vi "Terminal-GearSystem-Getter20150815.vi"(8 "error in (no error)":errorcluster caption="错误输入（无错误）", 11 "read operation timeout (ms)":i32=5000 caption="读操作超时（5000毫秒）") -> (0 "error out":errorcluster caption="错误输出", 2 "时间标识":timestamp, 3 "设备信息":T1)   [LabVIEW 2014]
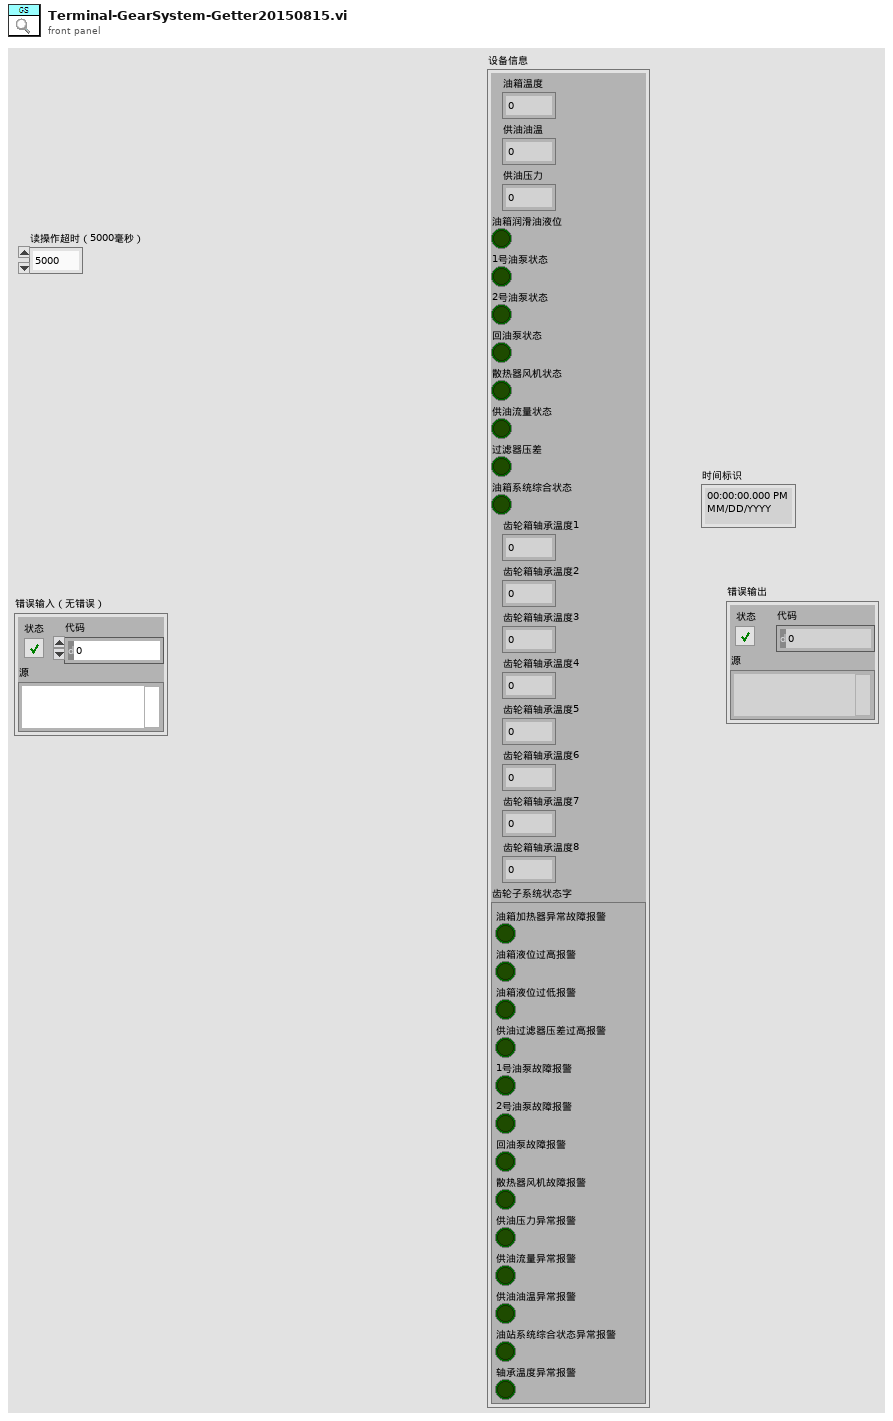
[diagram p1: front panel]
types:
  T1 = cluster{"油箱温度":u16, "供油油温":u16, "供油压力":u16, "油箱润滑油液位":bool, "1号油泵状态":bool, "2号油泵状态":bool, "回油泵状态":bool, "散热器风机状态":bool, "供油流量状态":bool, "过滤器压差":bool, "油箱系统综合状态":bool, "齿轮箱轴承温度1":u16, "齿轮箱轴承温度2":u16, "齿轮箱轴承温度3":u16, "齿轮箱轴承温度4":u16, "齿轮箱轴承温度5":u16, "齿轮箱轴承温度6":u16, "齿轮箱轴承温度7":u16, "齿轮箱轴承温度8":u16, "齿轮子系统状态字":cluster{"油箱加热器异常故障报警":bool, "油箱液位过高报警":bool, "油箱液位过低报警":bool, "供油过滤器压差过高报警":bool, "1号油泵故障报警":bool, "2号油泵故障报警":bool, "回油泵故障报警":bool, "散热器风机故障报警":bool, "供油压力异常报警":bool, "供油流量异常报警":bool, "供油油温异常报警":bool, "油站系统综合状态异常报警":bool, "轴承温度异常报警":bool}}
  T2 = cluster{"油箱温度":u16, "供油油温":u16, "供油压力":u16, "油箱润滑油液位":u16, "1号油泵状态":u16, "2号油泵状态":u16, "回油泵状态":u16, "散热器风机状态":u16, "供油流量状态":u16, "过滤器压差":u16, "油箱系统综合状态":u16, "齿轮箱轴承温度1":u16, "齿轮箱轴承温度2":u16, "齿轮箱轴承温度3":u16, "齿轮箱轴承温度4":u16, "齿轮箱轴承温度5":u16, "齿轮箱轴承温度6":u16, "齿轮箱轴承温度7":u16, "齿轮箱轴承温度8":u16, "齿轮子系统状态字":cluster{"油箱加热器异常故障报警":bool, "油箱液位过高报警":bool, "油箱液位过低报警":bool, "供油过滤器压差过高报警":bool, "1号油泵故障报警":bool, "2号油泵故障报警":bool, "回油泵故障报警":bool, "散热器风机故障报警":bool, "供油压力异常报警":bool, "供油流量异常报警":bool, "供油油温异常报警":bool, "油站系统综合状态异常报警":bool, "轴承温度异常报警":bool}}
  T3 = cluster{"油箱加热器异常故障报警":bool, "油箱液位过高报警":bool, "油箱液位过低报警":bool, "供油过滤器压差过高报警":bool, "1号油泵故障报警":bool, "2号油泵故障报警":bool, "回油泵故障报警":bool, "散热器风机故障报警":bool, "供油压力异常报警":bool, "供油流量异常报警":bool, "供油油温异常报警":bool, "油站系统综合状态异常报警":bool, "轴承温度异常报警":bool}
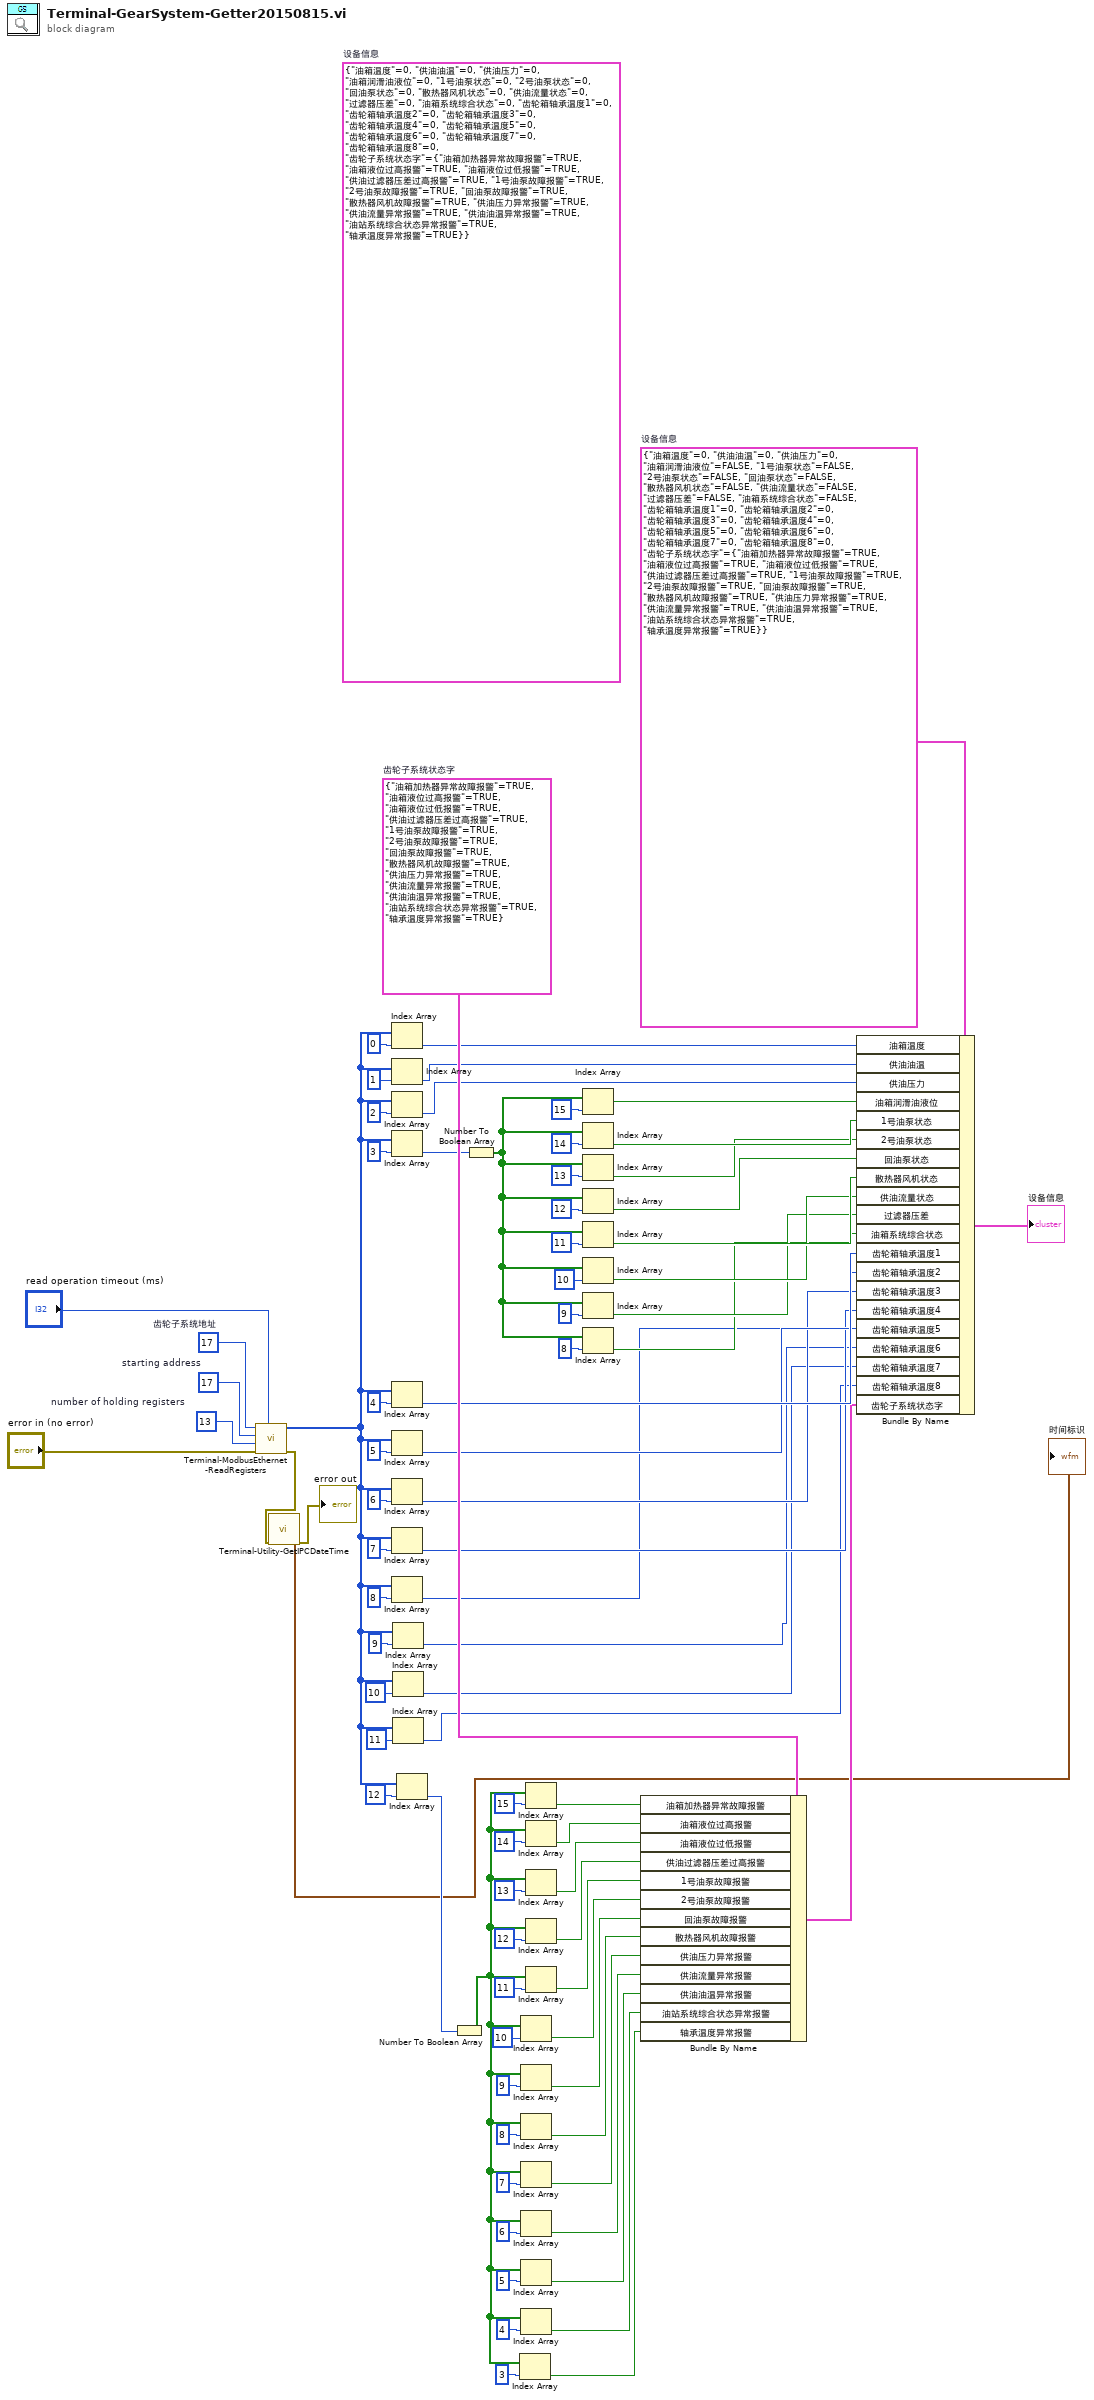
[diagram p0: block diagram]
diagram:
  (unwired) T2 {"油箱温度"=0, "供油油温"=0, "供油压力"=0, "油箱润滑油液位"=0, "1号油泵状态"=0, "2号油泵状态"=0, "回油泵状态"=0, "散热器风机状态"=0, "供油流量状态"=0, "过滤器压差"=0, "油箱系统综合状态"=0, "齿轮箱轴承温度1"=0, "齿轮箱轴承温度2"=0, "齿轮箱轴承温度3"=0, "齿轮箱轴承温度4"=0, "齿轮箱轴承温度5"=0, "齿轮箱轴承温度6"=0, "齿轮箱轴承温度7"=0, "齿轮箱轴承温度8"=0, "齿轮子系统状态字"={"油箱加热器异常故障报警"=TRUE, "油箱液位过高报警"=TRUE, "油箱液位过低报警"=TRUE, "供油过滤器压差过高报警"=TRUE, "1号油泵故障报警"=TRUE, "2号油泵故障报警"=TRUE, "回油泵故障报警"=TRUE, "散热器风机故障报警"=TRUE, "供油压力异常报警"=TRUE, "供油流量异常报警"=TRUE, "供油油温异常报警"=TRUE, "油站系统综合状态异常报警"=TRUE, "轴承温度异常报警"=TRUE}}  # 设备信息
  w42 = T3 {"油箱加热器异常故障报警"=TRUE, "油箱液位过高报警"=TRUE, "油箱液位过低报警"=TRUE, "供油过滤器压差过高报警"=TRUE, "1号油泵故障报警"=TRUE, "2号油泵故障报警"=TRUE, "回油泵故障报警"=TRUE, "散热器风机故障报警"=TRUE, "供油压力异常报警"=TRUE, "供油流量异常报警"=TRUE, "供油油温异常报警"=TRUE, "油站系统综合状态异常报警"=TRUE, "轴承温度异常报警"=TRUE}  # 齿轮子系统状态字
  w78 = T1 {"油箱温度"=0, "供油油温"=0, "供油压力"=0, "油箱润滑油液位"=FALSE, "1号油泵状态"=FALSE, "2号油泵状态"=FALSE, "回油泵状态"=FALSE, "散热器风机状态"=FALSE, "供油流量状态"=FALSE, "过滤器压差"=FALSE, "油箱系统综合状态"=FALSE, "齿轮箱轴承温度1"=0, "齿轮箱轴承温度2"=0, "齿轮箱轴承温度3"=0, "齿轮箱轴承温度4"=0, "齿轮箱轴承温度5"=0, "齿轮箱轴承温度6"=0, "齿轮箱轴承温度7"=0, "齿轮箱轴承温度8"=0, "齿轮子系统状态字"={"油箱加热器异常故障报警"=TRUE, "油箱液位过高报警"=TRUE, "油箱液位过低报警"=TRUE, "供油过滤器压差过高报警"=TRUE, "1号油泵故障报警"=TRUE, "2号油泵故障报警"=TRUE, "回油泵故障报警"=TRUE, "散热器风机故障报警"=TRUE, "供油压力异常报警"=TRUE, "供油流量异常报警"=TRUE, "供油油温异常报警"=TRUE, "油站系统综合状态异常报警"=TRUE, "轴承温度异常报警"=TRUE}}  # 设备信息
  w81 = u16 13  # number of holding registers
  w82 = u16 17  # starting address
  w83 = u8 17  # 齿轮子系统地址
  n1 = call "Terminal-ModbusEthernet-ReadRegisters.vi"("read operation timeout (ms)"="read operation timeout (ms)", "error in"="error in (no error)", "number of holding registers"=w81, "starting address"=w82, "unit ID"=w83) -> ("error out"=w2:errorcluster, "register values"=w17:u16[])  [unwired: 5 in]
  n2 = call "Terminal-Utility-GetIPCDateTime.vi"("error in (no error)"=w2) -> ("error out"=→"error out":errorcluster, "时间标识"=→"时间标识":timestamp)  [unwired: 9 in]
  n3 = Index Array(array=w17, index=0 ("索引")) -> (element=w41:u16)
  n4 = Index Array(array=w17, index=1 ("索引")) -> (element=w40:u16)
  n5 = Index Array(array=w17, index=2 ("索引")) -> (element=w39:u16)
  n6 = Index Array(array=w17, index=3 ("索引")) -> (element=w38:u16)
  n7 = Index Array(array=w17, index=4 ("索引")) -> (element=w16:u16)
  n8 = Index Array(array=w17, index=5 ("索引")) -> (element=w15:u16)
  n9 = Index Array(array=w17, index=6 ("索引")) -> (element=w14:u16)
  n10 = Index Array(array=w17, index=7 ("索引")) -> (element=w13:u16)
  n11 = Index Array(array=w17, index=8 ("索引")) -> (element=w12:u16)
  n12 = Index Array(array=w17, index=9 ("索引")) -> (element=w11:u16)
  n13 = Index Array(array=w17, index=10 ("索引")) -> (element=w10:u16)
  n14 = Index Array(array=w17, index=11 ("索引")) -> (element=w9:u16)
  n15 = Index Array(array=w17, index=12 ("索引")) -> (element=w73:u16)
  n16 = Number To Boolean Array(number=w73) -> (Boolean array=w7:bool[])
  n17 = Number To Boolean Array(number=w38) -> (Boolean array=w29:bool[])
  n18 = Index Array(array=w7, index=3 ("索引")) -> (element=w6:bool)
  n19 = Index Array(array=w7, index=10 ("索引")) -> (element=w49:bool)
  n20 = Index Array(array=w7, index=9 ("索引")) -> (element=w48:bool)
  n21 = Index Array(array=w7, index=8 ("索引")) -> (element=w47:bool)
  n22 = Index Array(array=w7, index=7 ("索引")) -> (element=w46:bool)
  n23 = Index Array(array=w7, index=6 ("索引")) -> (element=w43:bool)
  n24 = Index Array(array=w7, index=5 ("索引")) -> (element=w44:bool)
  n25 = Index Array(array=w7, index=4 ("索引")) -> (element=w45:bool)
  n26 = Index Array(array=w7, index=15 ("索引")) -> (element=w69:bool)
  n27 = Index Array(array=w7, index=14 ("索引")) -> (element=w68:bool)
  n28 = Index Array(array=w7, index=13 ("索引")) -> (element=w52:bool)
  n29 = Index Array(array=w7, index=12 ("索引")) -> (element=w51:bool)
  n30 = Index Array(array=w7, index=11 ("索引")) -> (element=w50:bool)
  n31 = Index Array(array=w29, index=15 ("索引")) -> (element=w28:bool)
  n32 = Index Array(array=w29, index=14 ("索引")) -> (element=w27:bool)
  n33 = Index Array(array=w29, index=13 ("索引")) -> (element=w26:bool)
  n34 = Index Array(array=w29, index=12 ("索引")) -> (element=w25:bool)
  n35 = Index Array(array=w29, index=11 ("索引")) -> (element=w24:bool)
  n36 = Index Array(array=w29, index=10 ("索引")) -> (element=w23:bool)
  n37 = Index Array(array=w29, index=9 ("索引")) -> (element=w22:bool)
  n38 = Index Array(array=w29, index=8 ("索引")) -> (element=w21:bool)
  n39 = Bundle By Name(cluster=w42, "油箱加热器异常故障报警"=w69, "油箱液位过高报警"=w68, "油箱液位过低报警"=w52, "供油过滤器压差过高报警"=w51, "1号油泵故障报警"=w50, "2号油泵故障报警"=w49, "回油泵故障报警"=w48, "散热器风机故障报警"=w47, "供油压力异常报警"=w46, "供油流量异常报警"=w43, "供油油温异常报警"=w44, "油站系统综合状态异常报警"=w45, "轴承温度异常报警"=w6) -> (w5:T3)
  n40 = Bundle By Name(cluster=w78, "油箱温度"=w41, "供油油温"=w40, "供油压力"=w39, "油箱润滑油液位"=w28, "1号油泵状态"=w27, "2号油泵状态"=w26, "回油泵状态"=w25, "散热器风机状态"=w24, "供油流量状态"=w23, "过滤器压差"=w22, "油箱系统综合状态"=w21, "齿轮箱轴承温度1"=w16, "齿轮箱轴承温度2"=w15, "齿轮箱轴承温度3"=w14, "齿轮箱轴承温度4"=w13, "齿轮箱轴承温度5"=w12, "齿轮箱轴承温度6"=w11, "齿轮箱轴承温度7"=w10, "齿轮箱轴承温度8"=w9, "齿轮子系统状态字"=w5) -> (→"设备信息":T1)
